vi "Pre-Build Action.vi"(6 "Top Level/Always Included VIs":path[](array[path]), 7 "Main Destination Path":path, 9 "Target Name":string, 10 "Build Specification Name":string, 11 "Project Path":path) -> (0 "error out":errorcluster)   [LabVIEW 2019]
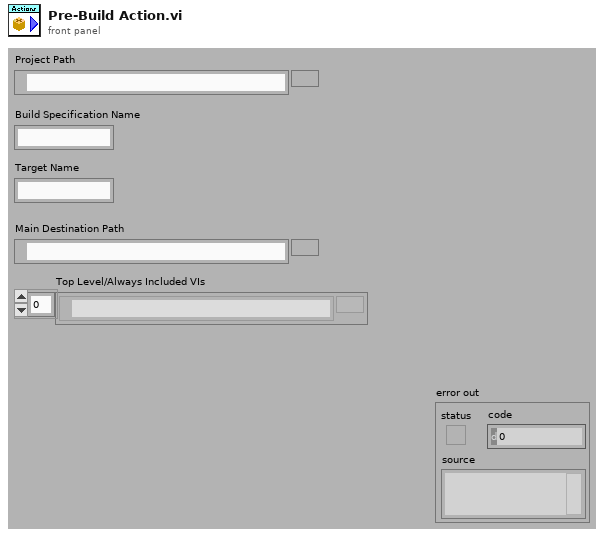
[diagram p1: front panel]
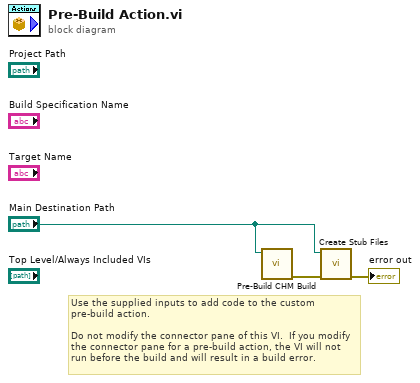
[diagram p0: block diagram]
diagram:
  # "Use the supplied inputs to add code to the custom pre-build action.\n\nDo not modify the connector pane of this VI.  If you modify the connector pane for a pre-build action, the VI will not run before the build and will result in a build error."
  n1 = call "Pre-Build CHM Build.vi"("Main Destination Path"="Main Destination Path") -> ("error out"=w3:errorcluster)  [unwired: 10 in]
  n2 = call "Create Stub Files.vi"("error in"=w3, "Main Destination Path"="Main Destination Path") -> ("error out"=→"error out":errorcluster)  [unwired: 9 in]
